vi "WM_CAP - Diagnostics Window.vi"(7 "CAPSTATUS In":T1) -> ()   [LabVIEW 2022 SP3]
panel:
  out "CAPSTATUS":T2
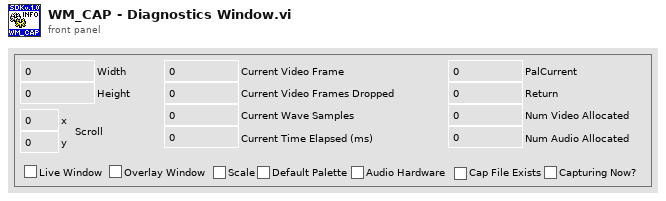
[diagram p1: front panel]
types:
  T1 = cluster{"uiImageWidth":u32, "uiImageHeight":u32, "fLiveWindow":u32, "fOverlayWindow":u32, "fScale":u32, "ptScroll":cluster{"x":i32, "y":i32}, "fUsingDefaultPalette":u32, "fAudioHardware":u32, "fCapFileExists":u32, "dwCurrentVideoFrame":u32, "dwCurrentVideoFramesDropped":u32, "dwCurrentWaveSamples":u32, "dwCurrentTimeElapsedMS":u32, "hPalCurrent":u32, "fCapturingNow":u32, "dwReturn":u32, "wNumVideoAllocated":u32, "wNumAudioAllocated":u32}
  T2 = cluster{"uiImageWidth":u32, "uiImageHeight":u32, "fLiveWindow":bool, "fOverlayWindow":bool, "fScale":bool, "ptScroll":cluster{"x":i32, "y":i32}, "fUsingDefaultPalette":bool, "fAudioHardware":bool, "fCapFileExists":bool, "dwCurrentVideoFrame":u32, "dwCurrentVideoFramesDropped":u32, "dwCurrentWaveSamples":u32, "dwCurrentTimeElapsedMS":u32, "hPalCurrent":u32, "fCapturingNow":bool, "dwReturn":u32, "wNumVideoAllocated":u32, "wNumAudioAllocated":u32}
  T3 = cluster{"uiImageWidth":u32, "uiImageHeight":u32, bool, bool, bool, "ptScroll":cluster{"x":i32, "y":i32}, bool, bool, bool, "dwCurrentVideoFrame":u32, "dwCurrentVideoFramesDropped":u32, "dwCurrentWaveSamples":u32, "dwCurrentTimeElapsedMS":u32, "hPalCurrent":u32, bool, "dwReturn":u32, "wNumVideoAllocated":u32, "wNumAudioAllocated":u32}
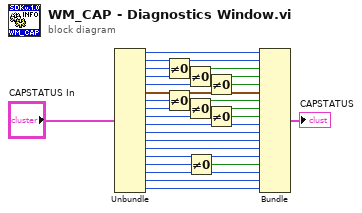
[diagram p0: block diagram]
diagram:
  n1 = Unbundle("CAPSTATUS In") -> ("uiImageWidth"=w3:u32, "uiImageHeight"=w12:u32, "fLiveWindow"=w13:u32, "fOverlayWindow"=w22:u32, "fScale"=w23:u32, "ptScroll"=w11:cluster{"x":i32, "y":i32}, "fUsingDefaultPalette"=w24:u32, "fAudioHardware"=w25:u32, "fCapFileExists"=w26:u32, "dwCurrentVideoFrame"=w10:u32, "dwCurrentVideoFramesDropped"=w9:u32, "dwCurrentWaveSamples"=w8:u32, "dwCurrentTimeElapsedMS"=w7:u32, "hPalCurrent"=w6:u32, "fCapturingNow"=w14:u32, "dwReturn"=w5:u32, "wNumVideoAllocated"=w4:u32, "wNumAudioAllocated"=w27:u32)
  n2 = Not Equal To 0?(x=w13) -> (x != 0?=w21:bool)
  n3 = Not Equal To 0?(x=w24) -> (x != 0?=w18:bool)
  n4 = Not Equal To 0?(x=w22) -> (x != 0?=w20:bool)
  n5 = Not Equal To 0?(x=w25) -> (x != 0?=w17:bool)
  n6 = Not Equal To 0?(x=w14) -> (x != 0?=w15:bool)
  n7 = Not Equal To 0?(x=w23) -> (x != 0?=w19:bool)
  n8 = Not Equal To 0?(x=w26) -> (x != 0?=w16:bool)
  n9 = Bundle("uiImageWidth"=w3, "uiImageHeight"=w12, w21, w20, w19, "ptScroll"=w11, w18, w17, w16, "dwCurrentVideoFrame"=w10, "dwCurrentVideoFramesDropped"=w9, "dwCurrentWaveSamples"=w8, "dwCurrentTimeElapsedMS"=w7, "hPalCurrent"=w6, w15, "dwReturn"=w5, "wNumVideoAllocated"=w4, "wNumAudioAllocated"=w27) -> (→"CAPSTATUS":T3)  [unwired: 1 in]
